vi "실습 9-5.vi"() -> ()   [LabVIEW 2014]
panel:
  out "웨이브폼 그래프":dbl[](graph)
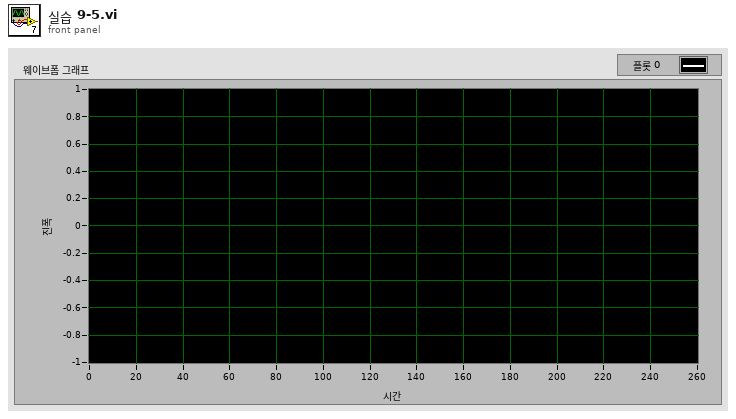
[diagram p1: front panel]
types:
  T1 = enum16{"big-endian, network order", "native, host order", "little-endian"}
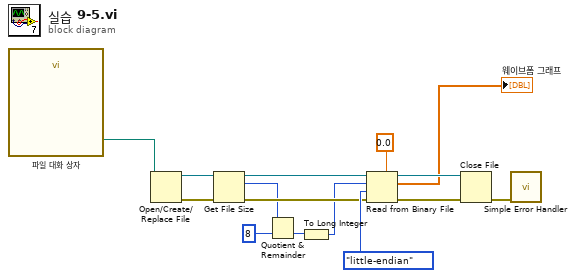
[diagram p0: block diagram]
diagram:
  n1 = call "파일 대화 상자"() -> ("selected path"=w1:path)  [unwired: 12 in, 3 out]
  n2 = Open/Create/Replace File(file path (use dialog)=w1) -> (refnum out=w10:refnum<file>, error out=w8:errorcluster)  [unwired: 5 in, 1 out]
  n3 = Get File Size(file=w10, error in=w8) -> (refnum out=w9:refnum<file>, size (in bytes)=w6:i64, 0:w7:errorcluster)
  n4 = Quotient & Remainder(x=w6, y=i64 8) -> (floor(x/y)=w4:i64)  [unwired: 1 out]
  n5 = To Long Integer(number=w4) -> (32bit integer=w3:i32)
  n6 = Read from Binary File(5:0.0, 8:w7, 9:T1."little-endian" ("바이트 순서(0:big-endian, network order)"), 10:w3, 11:w9) -> (0:w14:errorcluster, 2:→"웨이브폼 그래프":dbl[], 3:w15:refnum<file>)  [unwired: 1 in, 1 out]
  n7 = Close File(refnum=w15, error in=w14) -> (error out=w2:errorcluster)  [unwired: 1 out]
  n8 = call <vilib>:"Simple Error Handler.vi"("error in (no error)"=w2) -> ()  [unwired: 4 in, 5 out]
